vi "ref -- find member.vi"(7 "regexp":string="(\\s*[\\d\\.\\+\\-]+)+\\s*\\r?", 11 "save/read ref":refnum<vi>) -> (0 "Array":string[](array[string]), 1 "element":refnum<vi>, 2 "index":i32)   [LabVIEW 2018]
uses:
  freq file read-write control.ctl
panel:
  in  "save/read":T1={"write to a file list"=0, "from file "="1827_a", "erase"=FALSE, "load"=FALSE, "save"=FALSE, "to a file "="1827_a", "read from file list"=0} {"read from file list" items=["769_a", "841_a", "1399_a", "1502_a", "1527_a", "1705_a", "1916_a", "1958_a", "2061_a", "2227_a", "2365_a", "2551_a", "2713_a", "2761_a", "2964_a", "3000_a", "3030_a", "3084_a", "3235_a", "3366_a"]}
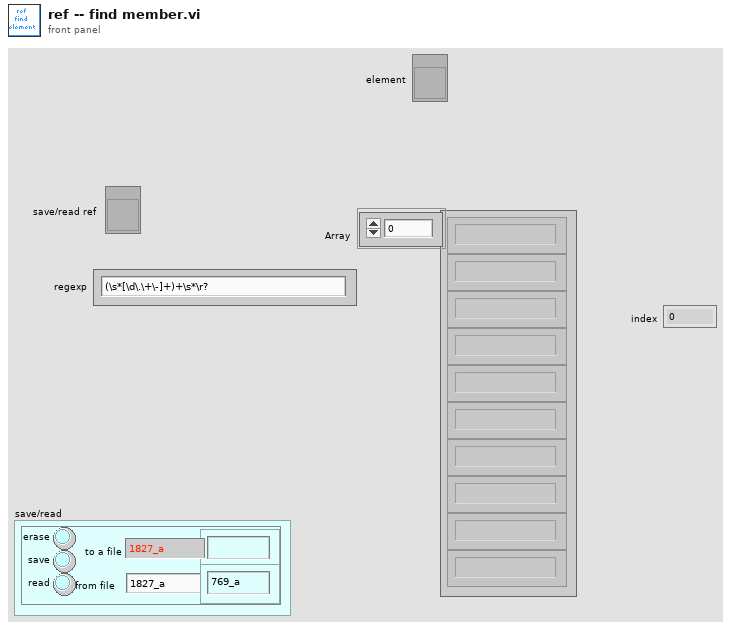
[diagram p1: front panel]
types:
  T1 = typedef "freq file read-write control.ctl" = cluster{"write to a file list":u16, "from file ":string, "erase":bool, "load":bool, "save":bool, "to a file ":string, "read from file list":u16}
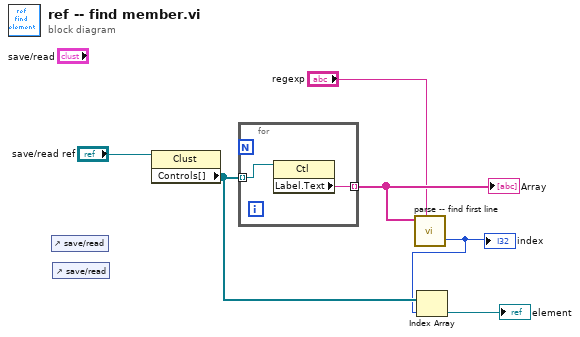
[diagram p0: block diagram]
diagram:
  n1 = control-ref of="save/read"() -> ()  [unwired: 1 out]
  n2 = control-ref of="save/read"() -> ()  [unwired: 1 out]
  n3 = property class="Clust"(reference="save/read ref") -> ("Controls[]"=w3:refnum<vi>[])  [unwired: 1 in, 2 out]
  n4 = for {
    tunnel: w3 -> [w8] mode=indexing
    tunnel: [w7] -> w6 mode=indexing
    n5 = property class="Ctl"(reference=w8) -> ("Label.Text"=w7:string)  [unwired: 1 in, 2 out]
  }
  "Array" <- w6
  n6 = call "parse -- find first line.vi"("regexp"="regexp", "string array"=w6) -> ("index"=w2:i32)  [unwired: 5 in, 4 out]
  "index" <- w2
  n7 = Index Array(array=w3, index=w2) -> (element=→"element":refnum<vi>)
